vi "ROI entry-Event handler-Max projection.vi"(8 "error in (no error)":errorcluster) -> (0 "error out":errorcluster)   [LabVIEW 2017]
uses:
  Typedefs/ROI management FG states.ctl
  ROI Entry screen/Globals/gl_ROI Entry UI globals.vi
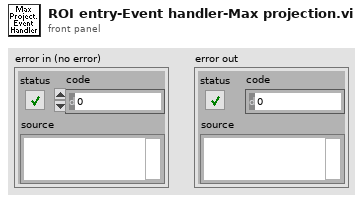
[diagram p1: front panel]
types:
  T1 = typedef "ROI entry screen ctrl refs cluster.ctl" = cluster{"Done button":refnum<vi>, "Imaging button":refnum<vi>, "Acquisition button":refnum<vi>, "POI dwell time (us)":refnum<vi>, "Scan dwell time per pixel (us)":refnum<vi>, "# of planes":refnum<vi>, "Zoom Ctrl":refnum<vi>, "Equal size":refnum<vi>, "Channel":refnum<vi>, "Image Display":refnum<vi>, "Z-Plane Selector":refnum<vi>, "Number of lines left":refnum<vi>, "Z-stack folder path":refnum<vi>, "POI Density":refnum<vi>, "Arb Plane Entry":refnum<vi>, "Whole plane":refnum<vi>, "Clear Last":refnum<vi>, "Clear All":refnum<vi>, "Trial Length (sec)":refnum<vi>, "Palette Type":refnum<vi>, "Intensity slider":refnum<vi>, "# POI":refnum<vi>, "Max Z Proj":refnum<vi>, "Zplane ind":refnum<vi>, "Wavelength (nm)":refnum<vi>, "Number of Trials":refnum<vi>, "Funct stim.trig.enable":refnum<vi>, "Funct stim.trig.delay (s)":refnum<vi>, "Line Mode":refnum<vi>, "Step size (µm)":refnum<vi>, "ROI move mode":refnum<vi>, "Cool-down time (s)":refnum<vi>, "Enable cool-down time":refnum<vi>, "Motor Z ind. (um)":refnum<vi>, "AOL Z ind. (um)":refnum<vi>, "Load Reference Image":refnum<vi>}
  T2 = typedef "ROI management FG states.ctl" = enum16{"Read", "Write", "Clear Last", "Clear All", "Update ROIs time", "Reload last ROI set", "Offset all ROI", "Offset visible ROI"}
  T3 = typedef "IMAQ Image.ctl" = refnum<image>
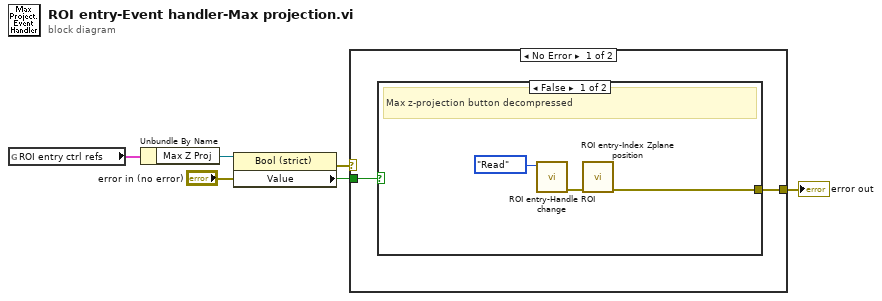
[diagram p0: block diagram]
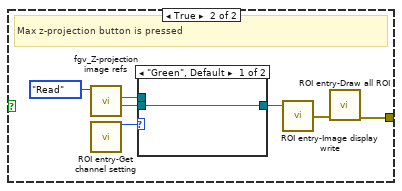
[diagram p2: hidden frame]
diagram:
  n1 = global read "gl_ROI Entry UI globals.vi" "ROI entry ctrl refs"() -> (w2:T1)
  n2 = Unbundle By Name(w2) -> ("Max Z Proj"=w3:refnum<vi>)
  n3 = property class="Bool (strict)"(reference=w3, error in="error in (no error)") -> (error out=w5:errorcluster, "Value"=w4:bool)  [unwired: 1 out]
  n4 = case shown="No Error" w5 {
    selector: w5 -> [_ w21]
    tunnel: w4 -> [w8 _]
    tunnel: [w7 w21] -> w6
    frame No Error {
      n5 = case shown="False" w8 {
        tunnel: [w9 w12] -> w7
        frame False {
          # "Max z-projection button decompressed"
          n6 = call "ROI entry-Handle ROI change.vi"("ROI management"=ROI_management_FG_states."Read" ("Function")) -> ("error out"=w11:errorcluster)  [unwired: 8 in, 2 out]
          n7 = call "ROI entry-Index Zplane position.vi"("error in (no error)"=w11) -> ("error out"=w9:errorcluster)  [unwired: 9 in, 1 out]
        }
        frame True {
          # "Max z-projection button is pressed"
          n8 = call "fgv_Z-projection image refs.vi"("Function"=enum16{"Intialize", "Write", "Read", "Clear"}."Read") -> ("GreenMaxZ"=w14:T3, "RedMaxZ"=w15:T3)  [unwired: 8 in, 1 out]
          n9 = call "ROI entry-Get channel setting.vi"() -> ("Selected channel"=w17:enum16{"Green", "Red"})  [unwired: 10 in, 1 out]
          n10 = case shown="\"Green\", Default" w17 {
            tunnel: [w19 w20] -> w18
            tunnel: w15 -> [_ w20]
            tunnel: w14 -> [w19 _]
            frame "Green", Default {
            }
            frame "Red" {
            }
          }
          n11 = call "ROI entry-Image display write.vi"("Value"=w18) -> ("error out"=w13:errorcluster)  [unwired: 4 in]
          n12 = call "ROI entry-Draw all ROI.vi"("error in (no error)"=w13) -> ("error out"=w12:errorcluster)  [unwired: 10 in]
        }
      }
    }
    frame Error {
    }
  }
  "error out" <- w6
